vi "Finish.vi"(8 "error in (no error)":errorcluster, 11 "Configuration File in":refnum<class "Configuration File.lvclass">) -> (0 "error out":errorcluster, 1 "Failed Keys":string[](array[string]), 2 "Failure (Errors or missing keys)?":bool, 3 "Configuration File out":refnum<class "Configuration File.lvclass">)   [LabVIEW 2018, in "Configuration File.lvlib" / "Configuration File.lvclass"]
doc: "This VI is used to close the reference to the configuration file.\n\nIT is recommended you open and close your config file in the code initialization, so you can replace it later in time while the code is running (especially since the code will de deployed as Run as Startup)"
uses:
  Configuration File.lvclass
  Configuration File.lvclass/Configuration File.ctl
  <vilib>/Utility/config.llb/NI_LVConfig.lvlib
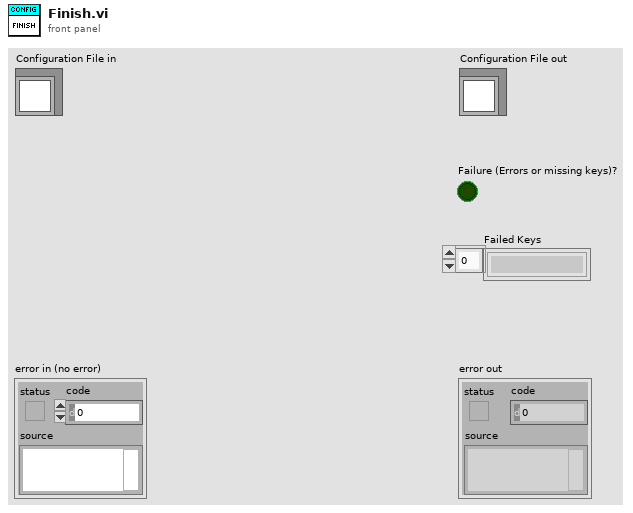
[diagram p1: front panel]
types:
  T1 = typedef "NI_LVConfig.lvlib/Config Data RefNum.ctl" = refnum<k1>
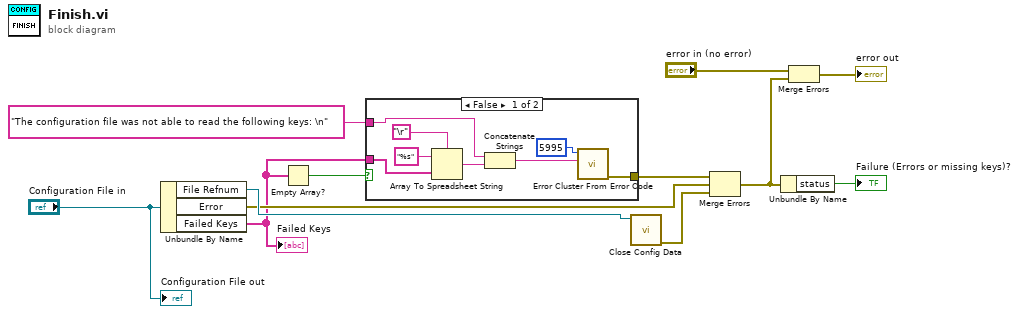
[diagram p0: block diagram]
diagram:
  n1 = Unbundle By Name("Configuration File in") -> ("File Refnum"=w10:T1, "Error"=w7:errorcluster, "Failed Keys"=w3:string[])
  "Failed Keys" <- w3
  n2 = Empty Array?(array=w3) -> (empty?=w5:bool)
  n3 = case shown="False" w5 {
    tunnel: [w20 _] -> w4
    tunnel: w3 -> [w17 _]
    tunnel: "The configuration file was not able to read the following keys: \n" ("error message (\"\")") -> [w13 _]
    frame False {
      n4 = Array To Spreadsheet String(delimiter (Tab)="\r", array=w17, 3:"%s" ("format string")) -> (spreadsheet string=w14:string)
      n5 = Concatenate Strings(w13, w14) -> (w18:string)
      n6 = call <vilib>:"Error Cluster From Error Code.vi"("error message (\"\")"=w18, "error code (0)"=5995) -> ("error out"=w20:errorcluster)  [unwired: 7 in]
    }
    frame True {
    }
  }
  n7 = call <vilib>:"Close Config Data.vi"("refnum"=w10) -> ("error out"=w8:errorcluster)  [unwired: 9 in, 1 out]
  n8 = Merge Errors(w4, w7, w8) -> (w1:errorcluster)
  n9 = Unbundle By Name(w1) -> ("status"=→"Failure (Errors or missing keys)?":bool)
  n10 = Merge Errors("error in (no error)", w1) -> (→"error out":errorcluster)
  "Configuration File out" <- "Configuration File in"
